vi "Create File.vi"(8 "error in (no error)":errorcluster) -> (0 "error out":errorcluster)   [LabVIEW 2010]
uses:
  Main/Main Globals.vi
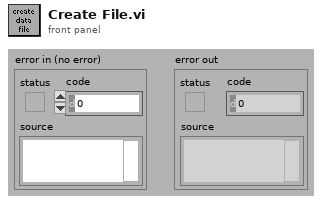
[diagram p1: front panel]
types:
  T1 = enum16{"open", "replace", "create", "open or create", "replace or create", "replace or create with confirmation"}
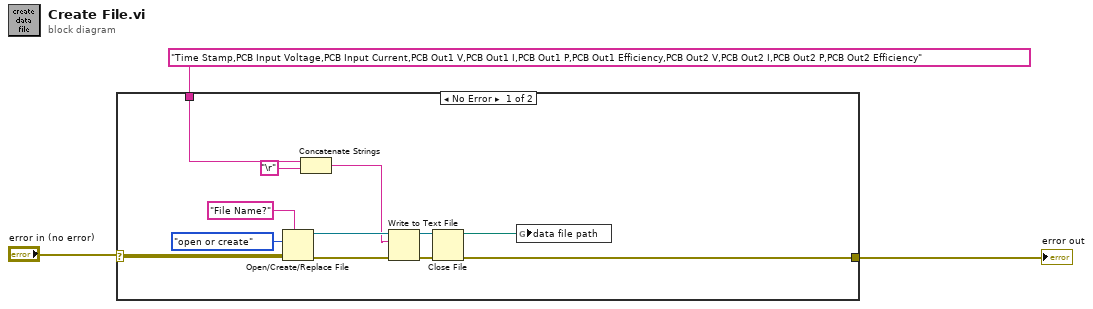
[diagram p0: block diagram]
diagram:
  n1 = case shown="No Error" "error in (no error)" {
    selector: "error in (no error)" -> [w15 w16]
    tunnel: [w4 w16] -> w2
    tunnel: "Time Stamp,PCB Input Voltage,PCB Input Current,PCB Out1 V,PCB Out1 I,PCB Out1 P,PCB Out1 Efficiency,PCB Out2 V,PCB Out2 I,PCB Out2 P,PCB Out2 Efficiency" ("format string") -> [w6 _]
    frame No Error {
      n2 = Open/Create/Replace File(error in=w15, prompt="File Name?", operation (0:open)=T1."open or create") -> (refnum out=w13:refnum<file>, error out=w14:errorcluster)  [unwired: 3 in, 1 out]
      n3 = Concatenate Strings(w6, "\r") -> (w7:string)
      n4 = Write to Text File(file (use dialog)=w13, text=w7, error in=w14) -> (refnum out=w11:refnum<file>, error out=w12:errorcluster)  [unwired: 1 in, 1 out]
      n5 = Close File(refnum=w11, error in=w12) -> (path=w5:path, error out=w4:errorcluster)
      n6 = global write "Main Globals.vi" "data file path"(w5) -> ()
    }
    frame Error {
    }
  }
  "error out" <- w2
